vi "Start Command.vi"(8 "error in (no error)":errorcluster, 11 "ReceiveCommand in":refnum<class "Announcing.lvclass">) -> (0 "error out":errorcluster, 3 "ReceiveCommand out":refnum<class "Announcing.lvclass">)   [LabVIEW 2013]
uses:
  Announcing.lvclass
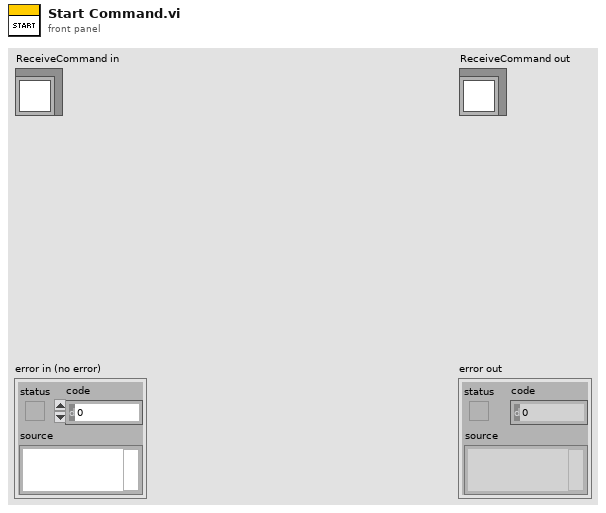
[diagram p1: front panel]
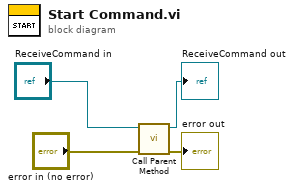
[diagram p0: block diagram]
diagram:
  n1 = call-parent "Call Parent Method"("error in (no error)"="error in (no error)", "ReceiveCommand in"="ReceiveCommand in") -> ("error out"=→"error out":errorcluster, "ReceiveCommand out"=→"ReceiveCommand out":refnum<class "Announcing.lvclass">)  [unwired: 8 in]
